vi "INIgetSection.vi"(10 "SectionName":string, 11 "INIfilePath":path) -> (0 "Error Out":errorcluster, 1 "SectionValues":string[](array[string]), 2 "SectionKeys":string[](array[string]))   [LabVIEW 2015]
uses:
  <vilib>/Utility/config.llb/Read Key (String).vi
  <vilib>/Utility/config.llb/NI_LVConfig.lvlib
panel:
  in  "Error In":errorcluster
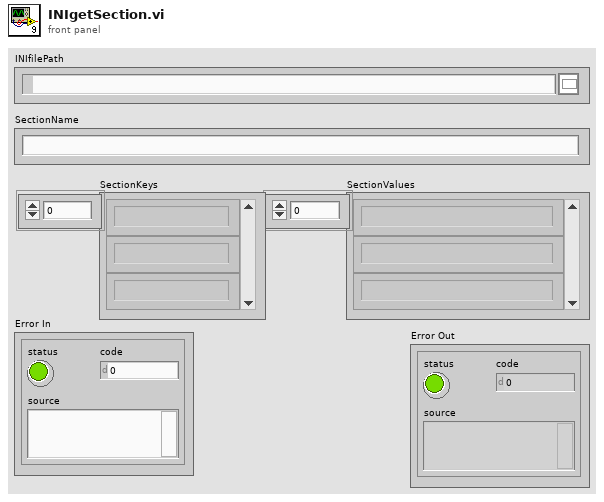
[diagram p1: front panel]
types:
  T1 = typedef "NI_LVConfig.lvlib/Config Data RefNum.ctl" = refnum<k1>
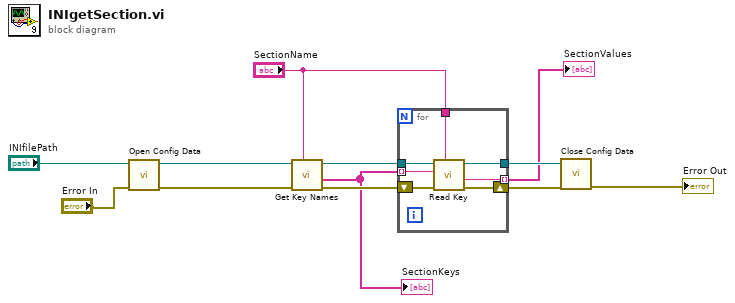
[diagram p0: block diagram]
diagram:
  n1 = call <vilib>:"Open Config Data.vi"("error in (no error)"="Error In", "configuration file path"="INIfilePath") -> ("error out"=w10:errorcluster, "refnum"=w12:T1)  [unwired: 7 in, 1 out]
  n2 = call <vilib>:"Get Key Names.vi"("section"="SectionName", "error in (no error)"=w10, "refnum"=w12) -> ("error out"=w4:errorcluster, "key names"=w1:string[], "refnum out"=w8:T1)  [unwired: 5 in, 1 out]
  "SectionKeys" <- w1
  n3 = for {
    tunnel: "SectionName" -> [w17]
    tunnel: w1 -> [w16] mode=indexing
    tunnel: w8 -> [w19]
    tunnel: [w18] -> w7
    tunnel: [w15] -> w5 mode=indexing
    shift-right: [w13] -> w3
    shift-left: w4 -> [w14]
    n4 = call-poly <vilib>:"Read Key.vi"("section"=w17, "error in (no error)"=w14, "key"=w16, "refnum"=w19) -> ("error out"=w13:errorcluster, "value"=w15:string, "refnum out"=w18:T1)  [unwired: 4 in, 1 out]
  }
  "SectionValues" <- w5
  n5 = call <vilib>:"Close Config Data.vi"("error in (no error)"=w3, "refnum"=w7) -> ("error out"=→"Error Out":errorcluster)  [unwired: 8 in, 1 out]
